vi "Parse.vi"(8 "Error In":errorcluster, 11 "object in":refnum<class "2025_2.lvclass">) -> (0 "Error Out":errorcluster, 3 "object out":refnum<class "2025_2.lvclass">)   [LabVIEW 2025, in "2025_2.lvclass"]
uses:
  2025_2.lvclass
  Range.ctl
  2025_2.lvclass/2025_2.ctl
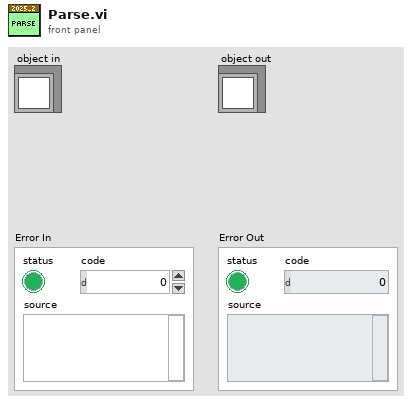
[diagram p1: front panel]
types:
  T1 = typedef "2025_2.lvclass/Range.ctl" = cluster{"Start":u64, "End":u64}
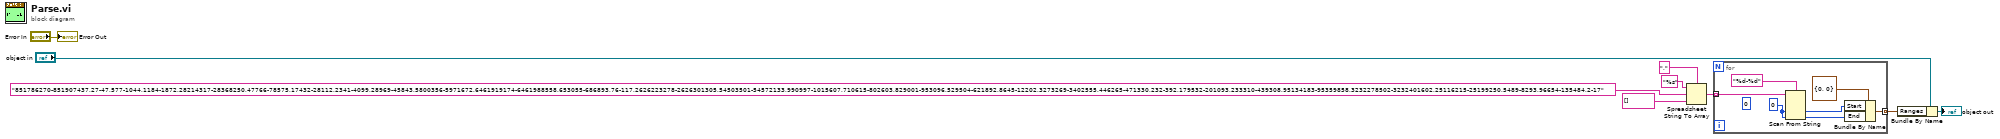
[diagram p0: block diagram]
diagram:
  n1 = Spreadsheet String To Array(delimiter (Tab)=",", format string="%s", spreadsheet string="851786270-851907437,27-47,577-1044,1184-1872,28214317-28368250,47766-78575,17432-28112,2341-4099,28969-45843,5800356-5971672,6461919174-6461988558,653055-686893,76-117,2626223278-2626301305,54503501-54572133,990997-1015607,710615-802603,829001-953096,529504-621892,8645-12202,3273269-3402555,446265-471330,232-392,179532-201093,233310-439308,95134183-95359858,3232278502-3232401602,25116215-25199250,5489-8293,96654-135484,2-17" ("PuzzleInput"), array type (2D Dbl)=string[] []) -> (array=w1:string[])
  n2 = for {
    tunnel: [w10] -> w6 mode=indexing
    tunnel: w1 -> [w16] mode=indexing
    w11 = u64 0 ("default value 14")
    (unwired) i64 0 ("default value 1")
    n3 = Scan From String(format string="%d-%d", input string=w16, default 1=w11, default 2=w11) -> (output 1=w14:u64, output 2=w13:u64)  [unwired: 2 in, 3 out]
    n4 = Bundle By Name(cluster=T1 {"Start"=0, "End"=0} ("Range"), "Start"=w14, "End"=w13) -> (w10:T1)
  }
  n5 = Bundle By Name(cluster="object in", "Ranges"=w6) -> (→"object out":refnum<class "2025_2.lvclass">)
  "Error Out" <- "Error In"
